vi "SowwahCX1.vi"(0 "Plot Array":cluster{dbl[], dbl[]}[](array[cluster])=[{[500.0, 500.0, 953.54, 215.0, 270.0, 320.0, 445.0, 525.0, 600.0, 675.0, 750.0, 825.0, 900.0, 960.0, 1010.0, 1060.0], [4.614524, 4.54365, 5.818368, 0.1374656, 0.6662545, 1.465458, 3.619824, 4.848976, 5.887329, 5.940571, 6.152151, 5.717487, 5.600293, 5.40069, 5.154843, 5.121789]}, {[100.0, 150.0, 215.0, 270.0, 320.0, 445.0, 525.0, 600.0, 675.0, 750.0, 825.0, 900.0, 960.0, 1010.0, 1060.0], [0.002314715, -0.00693192, 0.120417, 0.6880509, 1.519176, 3.513709, 5.065183, 6.116033, 6.096773, 5.938465, 5.593788, 5.5597, 5.387002, 5.304077, 4.887903]}] {"?" format="%.2f"; "?" format="%.2f"}, 1 "Job Directory":path=path "/G4_2_HD/Users/paulhayden/Documents/Projects/Westlakes_resolution") -> (2 "Saved Automatically?":bool, 3 "Tex Info String":string="set term epslatex\nset output \"Plot.eps\"\nset xlabel '$Distance~(m)$'\nset ylabel '$DF~(s/m^3)\\times10^6$'\nset samples 1000\nset pointsize 1.00\nset title '$B38~Centreline~Glc$' 0, 0\nset size 0.75,0.9\n\n#set key 450, -2.5833\n unset key\nset label 1 '~~~~~~~~~~~Angle~(deg)~=~0' at -100, -2.58\nset label 2 '~~~~~~~~~~~Height~(m)~=~5' at -100, -3.27\n set xrange [0 : 500] \n# set autoscale x \n set yrange [0.10000 : 7]\n# set autoscale y \n\nplot \"B38_Centreline_Glc.dat\" index 0 using 1:2 axes x1y1 title '$File=B38R~DDD.xls$' with points 1 1, \\\n\"B38_Centreline_Glc.dat\" index 1 using 1:2 axes x1y1 title '$File=B38R~DDD~1.xls$' with points 1 3", 4 "Plot data file":path)   [LabVIEW 2014]
uses:
  Results_plotter_Global.vi
panel:
  out "Output String":string
  out "subarray":string[](array[string])
  out "element":string
  out "Array":string[](array[string])
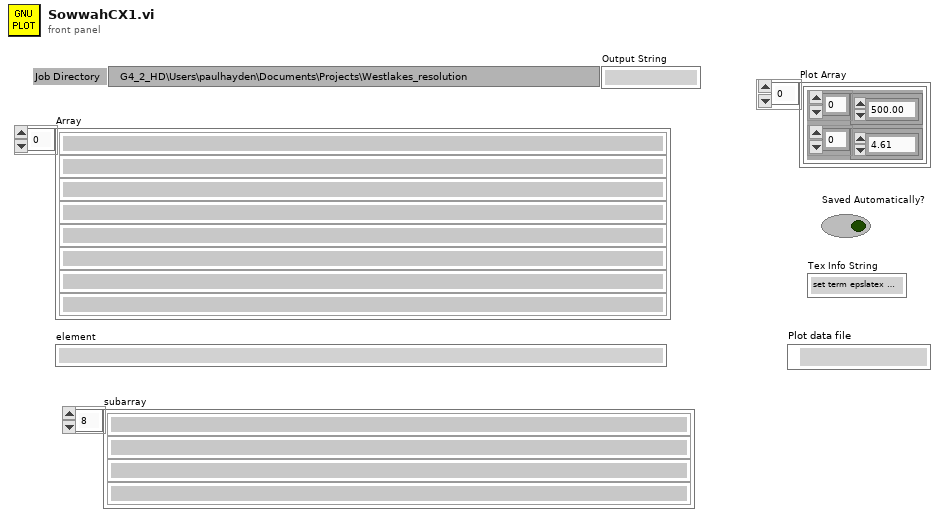
[diagram p1: front panel]
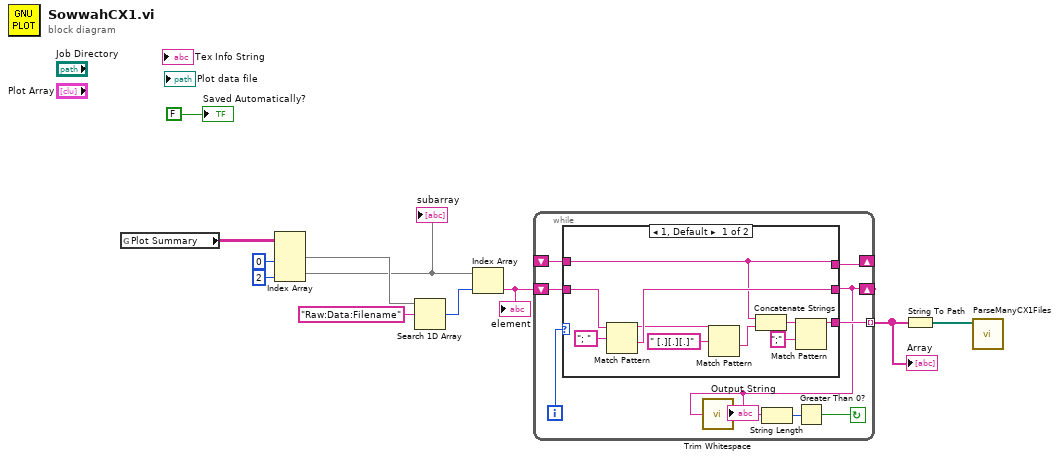
[diagram p0: block diagram]
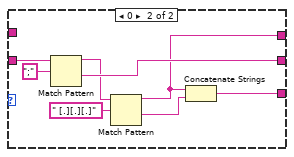
[diagram p2: hidden frame]
diagram:
  n1 = global read "Results_plotter_Global.vi" "Plot Summary"() -> (w10:string[][])
  n2 = Index Array(array=w10, index (col) #1=0 ("disabled index (col)"), index (col) #2=2 ("index (col)")) -> (element #1=w8:string[], element #2=w5:string[])  [unwired: 2 in]
  "subarray" <- w5
  n3 = Search 1D Array(1D array=w8, element="Raw:Data:Filename") -> (index of element=w4:i32)  [unwired: 1 in]
  n4 = Index Array(array=w5, index=w4) -> (element=w3:string)
  "element" <- w3
  n5 = while {
    tunnel: [w20] -> w1 mode=indexing
    shift-right: [w18] -> _
    shift-left: w3 -> [w19]
    shift-right: [w15] -> _
    shift-left: _ -> [w14]
    i -> [w13]
    stop <- w16 continue-if-true
    n6 = case shown="1, Default" w13 {
      tunnel: [w25 w31] -> w20
      tunnel: w19 -> [w29 w38]
      tunnel: [w28 w37] -> w18
      tunnel: [w27 w34] -> w15
      tunnel: w14 -> [w27 _]
      frame 1, Default {
        n7 = Match Pattern(string=w29, regular expression="; ") -> (before substring=w22:string, after substring=w28:string)  [unwired: 1 in, 2 out]
        n8 = Match Pattern(string=w22, regular expression=" [.][.][.]") -> (after substring=w21:string)  [unwired: 1 in, 3 out]
        n9 = Concatenate Strings(w27, w21) -> (w26:string)
        n10 = Match Pattern(string=w26, regular expression=";") -> (before substring=w25:string)  [unwired: 1 in, 3 out]
      }
      frame 0 {
        n11 = Match Pattern(string=w38, regular expression=";") -> (before substring=w36:string, after substring=w37:string)  [unwired: 1 in, 2 out]
        n12 = Match Pattern(string=w36, regular expression=" [.][.][.]") -> (before substring=w34:string, after substring=w33:string)  [unwired: 1 in, 2 out]
        n13 = Concatenate Strings(w34, w33) -> (w31:string)
      }
    }
    "Output String" <- w18
    n14 = call <vilib>:"Trim Whitespace.vi"("string"=w18) -> ("trimmed string"=w12:string)  [unwired: 1 in]
    n15 = String Length(string=w12) -> (length=w17:i32)
    n16 = Greater Than 0?(x=w17) -> (x > 0?=w16:bool)
  }
  "Array" <- w1
  n17 = String To Path(string=w1) -> (path=w2:path[])
  n18 = call "ParseManyCX1Files.vi"("Array"=w2) -> ()  [unwired: 11 in]
  "Saved Automatically?" <- FALSE
